vi "Simulate-Romi-Robot.vi"() -> ()   [LabVIEW 2020]
doc: "This WebSockets API example VI acts as a server for an incoming websockets connection. Receives/sends string data to the connected client."
uses:
  <vilib>/Rock Robotics/WPI/Simulation/Protocol/Devices/PWM/PWM proto.ctl
  <vilib>/Rock Robotics/WPI/Simulation/Protocol/Devices/PWM/PWM data proto.ctl
  <vilib>/Rock Robotics/WPI/Simulation/Protocol/Devices/RoboRIO/RoboRIO proto.ctl
  <vilib>/Rock Robotics/WPI/Simulation/Protocol/Devices/RoboRIO/RoboRIO data proto.ctl
  <vilib>/Rock Robotics/WPI/Simulation/Protocol/Devices/DriverStation/DS proto.ctl
  <vilib>/Rock Robotics/WPI/Simulation/Protocol/Devices/DriverStation/DS data proto.ctl
  <vilib>/Rock Robotics/WPI/Simulation/Protocol/Devices/DIO/DIO proto.ctl
  <vilib>/Rock Robotics/WPI/Simulation/Protocol/Devices/DIO/DIO data proto.ctl
  <vilib>/Rock Robotics/WPI/Simulation/Protocol/Devices/Gyro/Gyro proto.ctl
  <vilib>/Rock Robotics/WPI/Simulation/Protocol/Devices/Gyro/Gyro Data proto.ctl
  <vilib>/Rock Robotics/WPI/Simulation/Protocol/Devices/Encoder/Encoder proto.ctl
  <vilib>/Rock Robotics/WPI/Simulation/Protocol/Devices/Encoder/Encoder data protoo.ctl
  <vilib>/Rock Robotics/WPI/ThirdParty/JAS_Junk/TrajLib/DIFF_DRIVE_TRAIN_SIM.ctl
  <vilib>/Rock Robotics/WPI/ThirdParty/JAS_Junk/TrajLib/LINEAR_SYSTEM.ctl
  <vilib>/Analysis/Matrix/Datatypes/RealMatrix.ctl
  <vilib>/Rock Robotics/WPI/ThirdParty/JAS_Junk/TrajLib/DCMOTOR.CTL
  <vilib>/vision/Image Controls.llb/IMAQ Image.ctl
  ROBOT_PICTURE.ctl
  <vilib>/Utility/miscctls.llb/LVBoundsTypeDef.ctl
  <vilib>/Rock Robotics/SystemInterfaces/DIO/FPGA_DIOPWMChannel.ctl
  <vilib>/Rock Robotics/WPI/Simulation/Protocol/Devices/PWM/PWM Update Ops.ctl
  <vilib>/Rock Robotics/WPI/Simulation/Protocol/Devices/RoboRIO/RoboRIO Update Ops.ctl
  <vilib>/Rock Robotics/WPI/Simulation/Protocol/Devices/DriverStation/DS Update Ops.ctl
  <vilib>/Rock Robotics/SystemInterfaces/DIO/FPGA_DIOChannel.ctl
  <vilib>/Rock Robotics/WPI/Simulation/Protocol/Devices/DIO/DIO Update Ops.ctl
  <vilib>/Rock Robotics/WPI/Simulation/Protocol/Devices/Gyro/Gyro Update Ops.ctl
  <vilib>/Rock Robotics/WPI/Simulation/Protocol/Devices/Encoder/Encoder Update Ops.ctl
  <vilib>/Rock Robotics/SystemInterfaces/Encoder/FPGA_EncoderIdx.ctl
  <vilib>/Rock Robotics/WPI/ThirdParty/JAS_Junk/TrajLib/Rotation_CreateAngle.vi
  <vilib>/Rock Robotics/WPI/ThirdParty/JAS_Junk/TrajLib/Translation_Create.vi
  <vilib>/mediamongrels ltd/websockets/websockets/websocket server/websocket server.lvclass
  C:/Program Files (x86)/National Instruments/LabVIEW 2020/vi.lib/mediamongrels ltd/websockets/websockets/websocket/websocket.lvclass
  <vilib>/picture/pixmap.llb/Flatten Pixmap.vi
  <vilib>/picture/pictutil.llb/Create Mask.vi
  <vilib>/Rock Robotics/WPI/ThirdParty/JAS_Junk/TrajLib/Trajectory_Library.lvlib
  <vilib>/Analysis/Matrix/NI_Matrix.lvlib
panel:
  in  "Tab Control":T1(tab)
  in  "Button\n    C":bool
  in  "Button\n    B":bool
  out "Yellow LED":bool
  out "Green LED":bool
  out "Red LED":bool
  in  "Button\n    A":bool
  out "RSL ON":picture
  out "ROBOT":T2
  out "RSL OFF":picture
  out "Field Picture":picture
  out "Y Pos Pixel":dbl format="%11.1f"
  out "X Pos Pixel":dbl format="%11.1f"
  out "Y Pos Inch":dbl format="%11.1f"
  out "X Pos Inch":dbl format="%11.1f"
  out "Gyro":T3={"type"="AI", "device"="", "name"="", "data"={"<init"=FALSE, ">connected"=FALSE, "<offsetX"=0.0, "<offsetY"=0.0, "<offsetZ"=0.0, ">angleX"=0.0, ">angleY"=0.0, ">angleZ"=0.0, ">rateX"=0.0, ">rateY"=0.0, ">rateZ"=0.0, "<gain"=0.0}}
  out "DIO 0":T5={"type"="DIO", "device"="", "name"="", "data"={"<init"=FALSE, "<>value"=FALSE, "<pulse_length"=0, "<input"=FALSE}}
  out "Enc Left":T7={"type"="Encoder", "device"="", "name"="", "data"={"<init"=FALSE, ">count"=0.0, ">period"=0.0, "<samples_to_avg"=0, "<offset"=0.0, "<channel_a"=0, "<channel_b"=0}}
  out "Enc Right":T7={"type"="Encoder", "device"="", "name"="", "data"={"<init"=FALSE, ">count"=0.0, ">period"=0.0, "<samples_to_avg"=0, "<offset"=0.0, "<channel_a"=0, "<channel_b"=0}}
  out "DIO 1\nIn":T5={"type"="DIO", "device"="", "name"="", "data"={"<init"=FALSE, "<>value"=FALSE, "<pulse_length"=0, "<input"=FALSE}}
  out "DIO 2\nIn":T5={"type"="DIO", "device"="", "name"="", "data"={"<init"=FALSE, "<>value"=FALSE, "<pulse_length"=0, "<input"=FALSE}}
  out "PWM 0":T9
  out "PWM 1":T9
  out "DIO 1\nOut":T5={"type"="DIO", "device"="", "name"="", "data"={"<init"=FALSE, "<>value"=FALSE, "<pulse_length"=0, "<input"=FALSE}}
  out "DIO 2\nOut":T5={"type"="DIO", "device"="", "name"="", "data"={"<init"=FALSE, "<>value"=FALSE, "<pulse_length"=0, "<input"=FALSE}}
  out "DIO 3":T5={"type"="DIO", "device"="", "name"="", "data"={"<init"=FALSE, "<>value"=FALSE, "<pulse_length"=0, "<input"=FALSE}}
  out "roboRIO new":T11={"type"="roboRIO", "device"="", "name"="", "data"={">fpga_button"=FALSE, ">vin_voltage"=0.0, ">vin_current"=0.0, ">6v_voltage"=0.0, ">6v_current"=0.0, ">6v_active"=FALSE, ">6v_faults"=0.0, ">5v_voltage"=0.0, ">5v_current"=0.0, ">5v_active"=FALSE, ">5v_faults"=0.0, ">3v3_voltage"=0.0, ">3v3_current"=0.0, ">3v3_active"=FALSE, ">3v3_faults"=0.0}}
  out "Driverstation new":T13={"type"="Driverstation", "device"="", "name"="", "data"={">enabled"=FALSE, ">autonomous"=FALSE, ">test"=FALSE, ">estop"=FALSE, ">fms"=FALSE, ">ds"=FALSE, "<match_time"=0.0, ">station"="", ">game_data"=""}}
  out "Request URI":string
  out "HTTP Headers":variant
  out "Stop Sim":bool
  out "Battery Voltage VDC":dbl format="%18.2f"
  out "Sim Heading":dbl format="%19.3f"
  out "Edges/Feet":dbl
  out "out DiffDriveTrainSim":T15 {"m_Motor"."Jr_KgM2" format="%13.5p"; "m_Motor"."L_H" format="%13.5p"; "m_Motor"."Kt_NMPerAmp" format="%13.5p"; "m_Motor"."KvINV_RadPerSecPerVolt" format="%13.5p"; "m_Motor"."R_Ohms" format="%13.5p"; "m_Motor"."FreeSpeed_RadPerSec" format="%13.5p"; "m_Motor"."FreeCurrent_Amps" format="%13.5p"; "m_Motor"."StallCurrent_Amps" format="%13.5p"; "m_Motor"."StallTorque_NM" format="%13.5p"; "m_Motor"."nominalVoltage_Volts" format="%13.5p"}
  out "Speed Left":dbl format="%13.2f"
  out "Speed Right":dbl format="%13.2f"
  out "Amps":dbl
  out "PWM 0 Rate":dbl format="%19.3f"
  out "PWM 1 Rate":dbl format="%19.3f"
  out "FIeld Image":T19
  # "Robot Position"
  # "<States, 1>"
  # "<Outputs, 1>"
  # "<Inputs, 1>"
  # "<Outputs, 1>"
  # "<States,States>"
  # "<States,Inputs>"
  # "<Outputs,States>"
  # "<Outputs,Inputs>"
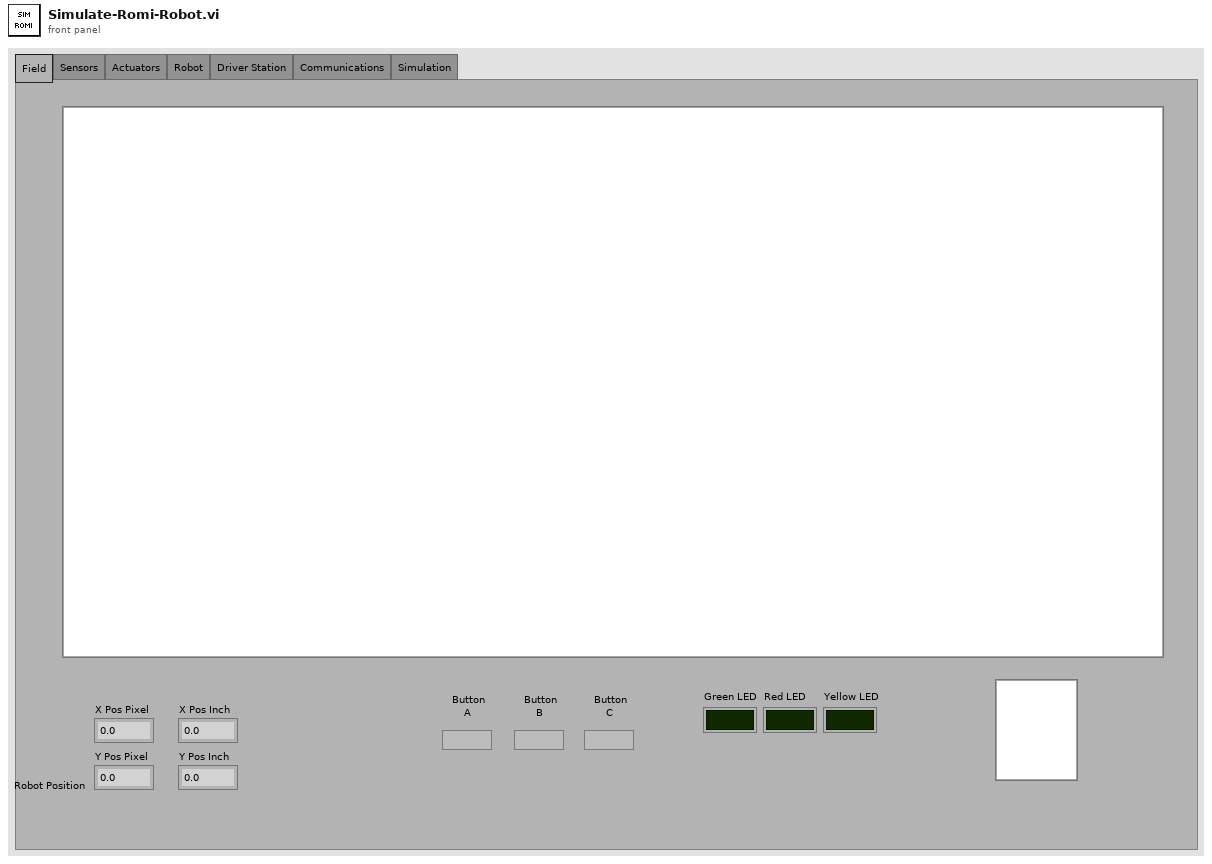
[diagram p1: front panel]
types:
  T1 = enum32{"Field", "Sensors", "Actuators", "Robot", "Driver Station", "Communications", "Simulation"}
  T2 = typedef "ROBOT_PICTURE.ctl" = picture
  T3 = typedef "Gyro proto.ctl" = cluster{"type":string, "device":string, "name":string, "data":T4}
  T4 = typedef "Gyro Data proto.ctl" = cluster{"<init":bool, ">connected":bool, "<offsetX":dbl, "<offsetY":dbl, "<offsetZ":dbl, ">angleX":dbl, ">angleY":dbl, ">angleZ":dbl, ">rateX":dbl, ">rateY":dbl, ">rateZ":dbl, "<gain":dbl}
  T5 = typedef "DIO proto.ctl" = cluster{"type":string, "device":string, "name":string, "data":T6}
  T6 = typedef "DIO data proto.ctl" = cluster{"<init":bool, "<>value":bool, "<pulse_length":i32, "<input":bool}
  T7 = typedef "Encoder proto.ctl" = cluster{"type":string, "device":string, "name":string, "data":T8}
  T8 = typedef "Encoder data protoo.ctl" = cluster{"<init":bool, ">count":dbl, ">period":dbl, "<samples_to_avg":i32, "<offset":dbl, "<channel_a":i32, "<channel_b":i32}
  T9 = typedef "PWM proto.ctl" = cluster{"type":string, "device":string, "name":string, "data":T10}
  T10 = typedef "PWM data proto.ctl" = cluster{"<init":bool, "<speed":dbl, "<position":dbl, "<raw":dbl, "<period_scale":dbl, "<zero_latch":bool, "<servo range":dbl}
  T11 = typedef "RoboRIO proto.ctl" = cluster{"type":string, "device":string, "name":string, "data":T12}
  T12 = typedef "RoboRIO data proto.ctl" = cluster{">fpga_button":bool, ">vin_voltage":dbl, ">vin_current":dbl, ">6v_voltage":dbl, ">6v_current":dbl, ">6v_active":bool, ">6v_faults":dbl, ">5v_voltage":dbl, ">5v_current":dbl, ">5v_active":bool, ">5v_faults":dbl, ">3v3_voltage":dbl, ">3v3_current":dbl, ">3v3_active":bool, ">3v3_faults":dbl}
  T13 = typedef "DS proto.ctl" = cluster{"type":string, "device":string, "name":string, "data":T14}
  T14 = typedef "DS data proto.ctl" = cluster{">enabled":bool, ">autonomous":bool, ">test":bool, ">estop":bool, ">fms":bool, ">ds":bool, "<match_time":dbl, ">station":string, ">game_data":string}
  T15 = typedef "Trajectory_Library.lvlib/DIFF_DRIVE_TRAIN_SIM.ctl" = cluster{"m_Plant":T16, "m_X":T17, "m_Y":T17, "m_U":T17, "MeasureStdDev":T17, "m_Motor":T18, "m_OriginalGearing":dbl, "m_CurrentGearing":dbl, "m_WheelRadius_M":dbl, "m_RB":dbl}
  T16 = typedef "Trajectory_Library.lvlib/LINEAR_SYSTEM.ctl" = cluster{"m_A":T17, "m_B":T17, "m_C":T17, "m_D":T17, "States":i32, "Inputs":i32, "Outputs":i32}
  T17 = typedef "NI_Matrix.lvlib/RealMatrix.ctl" = dbl[][]
  T18 = typedef "Trajectory_Library.lvlib/DCMOTOR.CTL" = cluster{"nominalVoltage_Volts":dbl, "StallTorque_NM":dbl, "StallCurrent_Amps":dbl, "FreeCurrent_Amps":dbl, "FreeSpeed_RadPerSec":dbl, "R_Ohms":dbl, "KvINV_RadPerSecPerVolt":dbl, "Kt_NMPerAmp":dbl, "L_H":dbl, "Jr_KgM2":dbl}
  T19 = typedef "IMAQ Image.ctl" = refnum<image>
  T20 = typedef "LVBoundsTypeDef.ctl" = cluster{"Width":u32, "Height":u32}
  T21 = typedef "Image Type" = u32
  T22 = typedef "imagedata.ctl" = cluster{"image type":i32, "image depth":i32, "image":u8[], "mask":u8[], "colors":u32[], "Rectangle":cluster{"left":i16, "top":i16, "right":i16, "bottom":i16}}
  T23 = typedef "TrajectoryUtils_Field_Info.ctl" = cluster{"FIeld_File_Name":string, "Top_Left_X":i32, "Top_Left_Y":i32, "Bottom_Right_X":i32, "Bottom_Right_Y":i32, "Field_Size_X":dbl, "Field_Size_Y":dbl, "FIeld_Size_Units":string}
  T24 = typedef "Trajectory_Library.lvlib/POSE2D.ctl" = cluster{"TRANSLATION":T25, "ROTATION":T26}
  T25 = typedef "Trajectory_Library.lvlib/TRANSLATION2D.ctl" = cluster{"X":dbl, "Y":dbl}
  T26 = typedef "Trajectory_Library.lvlib/ROTATION2D.ctl" = cluster{"VALUE":dbl, "COS":dbl, "SIN":dbl}
  T27 = typedef "Rotated_Picture_TypeDef.ctl" = cluster{"ONE-8-bit pixmap":u8[][], "Two-Array":cdb[][], "Three-Numeric":i32, "Four-Numeric":i32, "Five-Numeric":cdb, "Six-colors":u32[], "Seven-new element/subarray":u32, "Eight-Cluster":cluster{"[0]":i32, "[1]":i32}}
  T28 = typedef "Encoder Update Ops.ctl" = enum16{"set init", "set count", "set period", "set reset", "set samples_to_avg", "get", "delete", "JSON update", "set name", "transmit initial", "reset", "set channel_a", "set channel_b"}
  T29 = typedef "FPGA_EncoderIdx.ctl" = enum8{"Enc 0", "Enc 1", "Enc 2", "Enc 3", "Enc 4", "Enc 5", "Enc 6", "Enc 7", "Invalid"}
  T30 = typedef "Gyro Update Ops.ctl" = enum16{"get", "delete", "JSON update", "set  name", "transmit initial", "reset", "set init", "set offsetX", "set offsetY", "set offsetZ", "set gain"}
  T31 = typedef "FPGA_DIOChannel.ctl" = enum8{"DIO 0", "DIO 1", "DIO 2", "DIO 3", "DIO 4", "DIO 5", "DIO 6", "DIO 7", "DIO 8", "DIO 9", "DIO MXP 0", "DIO MXP 1", "DIO MXP 2", "DIO MXP 3", "DIO MXP 4", "DIO MXP 5", "DIO MXP 6", "DIO MXP 7", "DIO MXP 8", "DIO MXP 9", "DIO MXP 10", "DIO MXP 11", "DIO MXP 12", "DIO MXP 13", "DIO MXP 14", "DIO MXP 15", "SPI Port CS1", "SPI Port CS2", "SPI Port CS3", "SPI Port MISO", "SPI Port MOSI", "Invalid"}
  T32 = typedef "DIO Update Ops.ctl" = enum16{"set init", "set value", "set pulse_length", "set input", "get", "delete", "JSON update", "set name", "transmit initial", "reset"}
  T33 = typedef "DS Update Ops.ctl" = enum16{"set enabled", "set autonomous", "set test", "set estop", "set fms", "set ds", "set control word", "set match_time", "set station", "set game data", "JSON update", "set name", "get", "transmit initial", "reset"}
  T34 = typedef "RoboRIO Update Ops.ctl" = enum16{"get", "JSON update", "set name", "transmit initial", "set fpga_button", "set vin_voltage", "set vin_current", "set 6v_voltage", "set 6v_current", "set 6v_active", "set 6v_faults", "set 5v_voltage", "set 5v_current", "set 5v_active", "set 5v_faults", "set 3v3_voltage", "set 3v3_current", "set 3v3_active", "set 3v3_faults", "reset"}
  T35 = typedef "FPGA_DIOPWMChannel.ctl" = enum8{"PWM 0", "PWM 1", "PWM 2", "PWM 3", "PWM 4", "PWM 5", "PWM 6", "PWM 7", "PWM 8", "PWM 9", "PWM MXP 0", "PWM MXP 1", "PWM MXP 2", "PWM MXP 3", "PWM MXP 4", "PWM MXP 5", "PWM MXP 6", "PWM MXP 7", "PWM MXP 8", "PWM MXP 9", "Invalid"}
  T36 = typedef "PWM Update Ops.ctl" = enum16{"set init", "set speed", "set position", "set raw", "set  period_scale", "set zero_latch", "set angular range", "get", "delete", "JSON update", "set name", "transmit initial", "reset"}
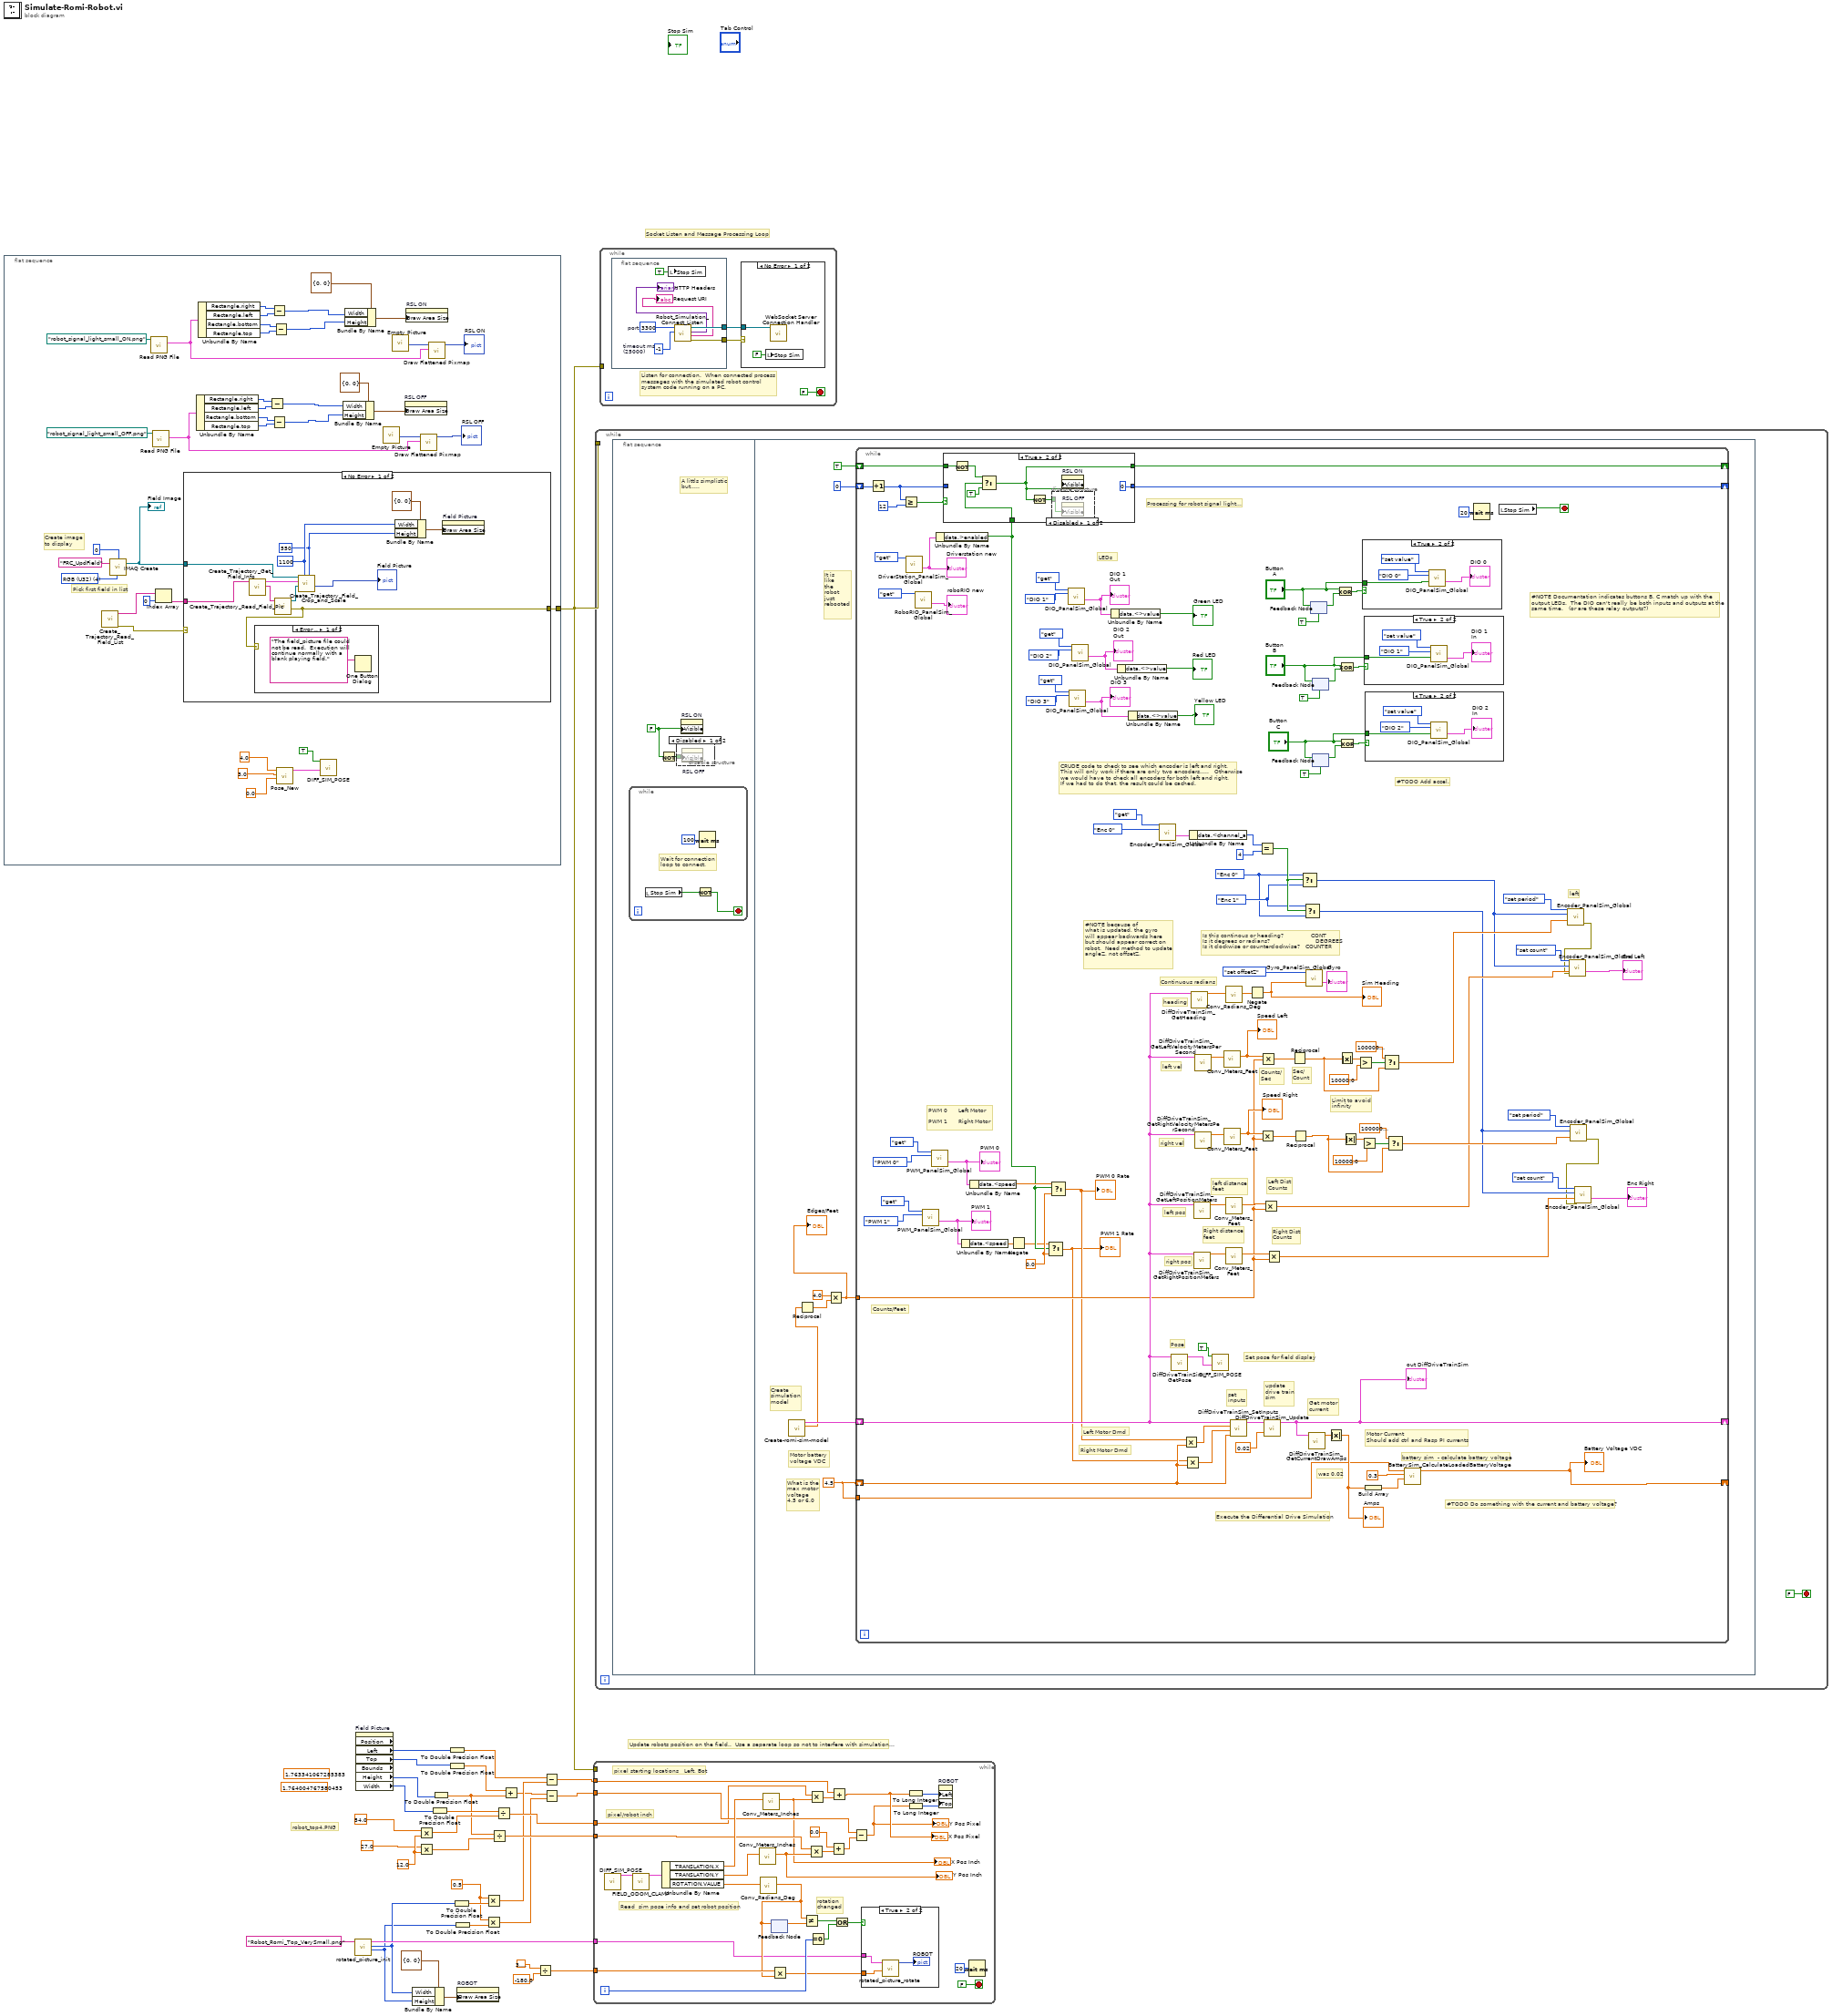
[diagram p0: block diagram]
diagram:
  w9 = 0.5
  (unwired) 1.764004767580453
  (unwired) 1.763341067285383
  w27 = 12.0 ("y")
  # "Update robots position on the field..  Use a separate loop so not to interfere with simulation..."
  # "robot_top4.PNG"
  # "Socket Listen and Message Processing Loop"
  n1 = flat-sequence {
    tunnel: [w43] -> w28
    frame #0 {
      w68 = T21 4 items=["Grayscale (U8)", "Grayscale (I16)", "Grayscale (SGL)", "Complex (CSG)", "RGB (U32)", "HSL (U32)", "RGB (U64)", "Grayscale (U16)"] ("Image Type")
      # "Pick first field in list"
      # "Create image \nto display"
      n2 = call "Create_Trajectory_Read_Field_List.vi"() -> ("error out"=w66:errorcluster, "section names"=w67:string[])  [unwired: 10 in]
      n3 = call "IMAQ Create"("Border Size"=0, "Image Name"="FRC_UpdField", "Image Type"=w68) -> ("New Image"=w65:T19)  [unwired: 2 in, 1 out]
      "FIeld Image" <- w65
      n4 = call <vilib>:"Read PNG File.vi"("path to PNG file"=path "robot_signal_light_small_ON.png") -> ("image data"=w54:T22)  [unwired: 8 in, 2 out]
      n5 = call <vilib>:"Read PNG File.vi"("path to PNG file"=path "robot_signal_light_small_OFF.png") -> ("image data"=w61:T22)  [unwired: 8 in, 2 out]
      n6 = Index Array(array=w67, index=0) -> (element=w64:string)
      n7 = case shown="No Error" w66 {
        selector: w66 -> [_ w84]
        tunnel: w65 -> [w79 _]
        tunnel: [w78 w84] -> w43
        tunnel: w64 -> [w77 _]
        frame No Error {
          w72 = 550 ("Disp Y Size Pixel")
          w73 = 1100 ("Disp X Size Pixel")
          n8 = call "Create_Trajectory_Get_Field_Info.vi"("Field Selector"=w77) -> ("File"=w82:string, "input cluster"=w81:T23)  [unwired: 9 in]
          n9 = call "Create_Trajectory_Read_Field_Pic.vi"("file name"=w82) -> ("Image Error"=w78:errorcluster, "Image Data"=w80:T19)  [unwired: 7 in, 2 out]
          n10 = case shown="Error .." w78 {
            frame Error {
              n11 = One Button Dialog(message="The field_picture file could not be read.  Execution will continue normally with a blank playing field.") -> ()  [unwired: 1 in, 1 out]
            }
            frame No Error {
            }
          }
          n12 = call "Create_Trajectory_Field_Crop_and_Scale.vi"("Disp Y Size Pixel"=w72, "Disp X Size Pixel"=w73, "Field Image"=w80, "field Info"=w81, "Display Image"=w79) -> ("Cropped Field Picture Out"=→"Field Picture":picture)  [unwired: 4 in, 2 out]
          n13 = Bundle By Name(cluster=T20 {"Width"=0, "Height"=0} ("Draw Area Size"), "Width"=w73, "Height"=w72) -> (w74:T20)
          n14 = property on="Field Picture" class="Pict"("Draw Area Size"=w74) -> ()  [unwired: 2 in, 2 out]
        }
        frame Error {
        }
      }
      n15 = Unbundle By Name(w61) -> ("Rectangle.right"=w57:i16, "Rectangle.left"=w58:i16, "Rectangle.bottom"=w56:i16, "Rectangle.top"=w59:i16)
      n16 = Unbundle By Name(w54) -> ("Rectangle.right"=w49:i16, "Rectangle.left"=w50:i16, "Rectangle.bottom"=w48:i16, "Rectangle.top"=w51:i16)
      n17 = Subtract(x=w57, y=w58) -> (x-y=w35:i16)
      n18 = Subtract(x=w49, y=w50) -> (x-y=w37:i16)
      n19 = Subtract(x=w56, y=w59) -> (x-y=w34:i16)
      n20 = Subtract(x=w48, y=w51) -> (x-y=w36:i16)
      n21 = call <vilib>:"Pose_New.vi"("Heading"=0.0, "Y"=3.0, "X"=4.0) -> ("out POSe"=w41:T24)  [unwired: 8 in]
      n22 = call "DIFF_SIM_POSE.vi"("in Sim Pose"=w41, "WRITE"=TRUE) -> ()  [unwired: 9 in, 1 out]
      n23 = Bundle By Name(cluster=T20 {"Width"=0, "Height"=0} ("Draw Area Size"), "Width"=w35, "Height"=w34) -> (w63:T20)
      n24 = Bundle By Name(cluster=T20 {"Width"=0, "Height"=0} ("Draw Area Size"), "Width"=w37, "Height"=w36) -> (w52:T20)
      n25 = call "Empty Picture"() -> ("empty picture"=w60:picture)
      n26 = call "Empty Picture"() -> ("empty picture"=w53:picture)
      n27 = property on="RSL OFF" class="Pict"("Draw Area Size"=w63) -> ()  [unwired: 2 in, 2 out]
      n28 = property on="RSL ON" class="Pict"("Draw Area Size"=w52) -> ()  [unwired: 2 in, 2 out]
      n29 = call <vilib>:"Draw Flattened Pixmap.vi"("image data"=w61, "picture"=w60) -> ("new picture"=→"RSL OFF":picture)  [unwired: 7 in]
      n30 = call <vilib>:"Draw Flattened Pixmap.vi"("image data"=w54, "picture"=w53) -> ("new picture"=→"RSL ON":picture)  [unwired: 7 in]
    }
  }
  n31 = call "rotated_picture_init.vi"("Picture FIle Name"="Robot_Romi_Top_VerySmall.png" ("name or relative path")) -> ("Height"=w1:i16, "Width"=w2:i16, "RotatedPictureInfo"=w29:T27)  [unwired: 7 in, 1 out]
  n32 = property on="Field Picture" class="Pict" props=["Position", "Left", "Top", "Bounds", "Height", "Width"]() -> ("Left"=w24:i32, "Top"=w23:i32, "Height"=w22:u32, "Width"=w21:u32)  [unwired: 2 in, 4 out]
  n33 = Bundle By Name(cluster=T20 {"Width"=0, "Height"=0} ("Draw Area Size"), "Width"=w2, "Height"=w1) -> (w4:T20)
  n34 = Multiply(x=54.0, y=w27) -> (x*y=w18:dbl)
  n35 = Multiply(x=27.0, y=w27) -> (x*y=w15:dbl)
  n36 = To Double Precision Float(number=w21) -> (double precision float=w19:dbl)
  n37 = To Double Precision Float(number=w22) -> (double precision float=w16:dbl)
  n38 = To Double Precision Float(number=w24) -> (double precision float=w8:dbl)
  n39 = To Double Precision Float(number=w23) -> (double precision float=w20:dbl)
  n40 = To Double Precision Float(number=w2) -> (double precision float=w11:dbl)
  n41 = To Double Precision Float(number=w1) -> (double precision float=w10:dbl)
  n42 = property on="ROBOT" class="Pict (strict)"("Draw Area Size"=w4) -> ()  [unwired: 2 in, 2 out]
  n43 = Multiply(x=w9, y=w11) -> (x*y=w7:dbl)
  n44 = Multiply(x=w9, y=w10) -> (x*y=w5:dbl)
  n45 = Divide(x=w16, y=w15) -> (x/y=w14:dbl)
  n46 = Divide(x=w19, y=w18) -> (x/y=w17:dbl)
  n47 = Add(x=w20, y=w16) -> (x+y=w6:dbl)
  n48 = Divide(x=3.141592653589793, y=-180.0 ("value")) -> (x/y=w33:dbl)
  n49 = Subtract(x=w8, y=w7) -> (x-y=w13:dbl)
  n50 = Subtract(x=w6, y=w5) -> (x-y=w12:dbl)
  n51 = while {
    tunnel: w33 -> [w114]
    tunnel: w29 -> [w97]
    tunnel: w28 -> [_]
    tunnel: w13 -> [w94]
    tunnel: w12 -> [w93]
    tunnel: w17 -> [w92]
    tunnel: w14 -> [w91]
    i -> [w103]
    stop <- FALSE stop-if-true
    # "pixel starting locations   Left, Bot"
    # "Read  sim pose info and set robot position"
    # "pixel/robot inch"
    # "rotation\nchanged"
    n52 = call "DIFF_SIM_POSE.vi"() -> ("out Sim Pose"=w96:T24)  [unwired: 11 in]
    n53 = call "FIELD_ODOM_CLAMP.vi"("in Sim Pose"=w96) -> ("out Sim Pose"=w95:T24)  [unwired: 10 in]
    n54 = Unbundle By Name(w95) -> ("TRANSLATION.X"=w102:dbl, "TRANSLATION.Y"=w101:dbl, "ROTATION.VALUE"=w99:dbl)
    n55 = call <vilib>:"Conv_Meters_Inches.vi"("Meters"=w101) -> ("Inches"=w86:dbl)  [unwired: 10 in]
    "Y Pos Inch" <- w86
    n56 = call <vilib>:"Conv_Radians_Deg.vi"("Radians"=w99) -> ("Degrees"=w100:dbl)  [unwired: 10 in]
    n57 = call <vilib>:"Conv_Meters_Inches.vi"("Meters"=w102) -> ("Inches"=w85:dbl)  [unwired: 10 in]
    "X Pos Inch" <- w85
    n58 = feedback-in #1(w100) -> ()
    n59 = feedback #1() -> (w111:dbl)  [unwired: 1 in]
    n60 = Multiply(x=w114, y=w100) -> (x*y=w98:dbl)
    n61 = Not Equal?(x=w100, y=w111) -> (x != y?=w105:bool)
    n62 = Multiply(x=w91, y=w86) -> (x*y=w109:dbl)
    n63 = Multiply(x=w92, y=w85) -> (x*y=w110:dbl)
    n64 = Equal To 0?(x=w103) -> (x = 0?=w104:bool)
    n65 = Add(x=0.0, y=w109) -> (x+y=w107:dbl)
    n66 = Add(x=w94, y=w110) -> (x+y=w88:dbl)
    "X Pos Pixel" <- w88
    n67 = Or(x=w105, y=w104) -> (x .or. y?=w106:bool)
    n68 = Subtract(x=w93, y=w107) -> (x-y=w87:dbl)
    "Y Pos Pixel" <- w87
    n69 = case shown="True" w106 {
      tunnel: w98 -> [_ w115]
      tunnel: w97 -> [_ w116]
      frame False {
      }
      frame True {
        n70 = call "rotated_picture_rotate.vi"("Angle"=w115, "RotatedPictureInfo"=w116) -> ("new picture"=→"ROBOT":picture)  [unwired: 9 in]
      }
    }
    n71 = To Long Integer(number=w88) -> (32bit integer=w90:i32)
    n72 = To Long Integer(number=w87) -> (32bit integer=w89:i32)
    n73 = property on="ROBOT" class="Pict (strict)"("Left"=w90, "Top"=w89) -> ()  [unwired: 2 in, 2 out]
    n74 = Wait (ms)(milliseconds to wait=u32 20) -> ()  [unwired: 1 out]
  }
  n75 = while {
    tunnel: w28 -> [_]
    stop <- FALSE stop-if-true
    n76 = flat-sequence {
      frame #0 {
        w119 = FALSE ("Visible")
        # "A littls simplistic\nbut....."
        n77 = while {
          stop <- w122 stop-if-true
          # "Wait for connection\nloop to connect."
          n78 = local read "Stop Sim"() -> (w123:bool)
          n79 = Not(x=w123) -> (.not. x?=w122:bool)
          n80 = Wait (ms)(milliseconds to wait=u32 100) -> ()  [unwired: 1 out]
        }
        n81 = Not(x=w119) -> (.not. x?=w120:bool)
        n82 = disable-structure shown="Disabled" {
          disable-tunnel: w120 -> [w121 _]
          frame Disabled {
            n83 = property on="RSL OFF" class="Pict"("Visible"=w121) -> ()  [unwired: 2 in, 2 out]
          }
          frame Enabled {
          }
        }
        n84 = property on="RSL ON" class="Pict"("Visible"=w119) -> ()  [unwired: 2 in, 2 out]
      }
      frame #1 {
        w129 = 4.5 ("Voltage")
        # "Create\nsimulation\nmodel"
        # "Motor battery\nvoltage VDC"
        # "What is the\nmax motor\nvoltage\n4.5 or 6.0"
        # "It is\nlike\nthe \nrobot \njust\nrebooted"
        n85 = call "Create-romi-sim-model.vi"() -> ("Encoder Ft/Count"=w126:dbl, "out DiffDriveTrainSim"=w130:T15)  [unwired: 10 in]
        n86 = Reciprocal(x=w126) -> (1/x=w127:dbl)
        n87 = Multiply(x=4.0, y=w127) -> (x*y=w125:dbl)
        "Edges/Feet" <- w125
        n88 = while {
          shift-right: [w208] -> _
          shift-left: 0 -> [w213]
          shift-right: [w210] -> _
          shift-left: TRUE -> [w211]
          shift-right: [w191] -> _
          shift-left: w130 -> [w192]
          shift-right: [w188] -> _
          shift-left: w129 -> [w190]
          tunnel: w129 -> [w189]
          tunnel: w125 -> [w180]
          stop <- w215 stop-if-true
          w166 = FPGA_EncoderIdx."Enc 1" ("EncoderIndex")
          w165 = FPGA_EncoderIdx."Enc 0" ("EncoderIndex")
          w174 = 0.0 ("f")
          # "was 0.02"
          # "LEDs"
          # "#NOTE Documentation indicates buttons B, C match up with the\noutput LEDs.  The DIO can't really be both inputs and outputs at the\nsame time.   (or are these relay outputs?)"
          # "#NOTE because of\nwhat is updated, the gyro\nwill appear backwards here\nbut should appear correct on\nrobot.  Need method to update\nangleZ, not offsetZ."
          # "#TODO Add accel."
          # "left"
          # "CRUDE code to check to see which encoder is left and right.\nThis will only work if there are only two encoders.....   Otherwise\nwe would have to check all encoders for both left and right.\nIf we had to do that, the result could be cached."
          # "#TODO Do something with the current and battery voltage?"
          # "Right Dist\nCounts"
          # "Left Dist\nCounts"
          # "Is this continous or heading?               CONT\nIs it degrees or radians?                         DEGREES\nIs it clockwise or counterclockwise?   COUNTER"
          # "Sec/\nCount"
          # "Limit to avoid\ninfinity"
          # "Counts/\nSec"
          # "Counts/Feet"
          # "Get motor\ncurrent"
          # "Set pose for field display"
          # "PWM 0      Left Motor\n\nPWM 1      Right Motor"
          # "Motor Current\nShould add ctrl and Rasp PI currents"
          # "Right Motor Dmd"
          # "Left Motor Dmd"
          # "Continuous radians"
          # "Right distance\nfeet"
          # "left distance\nfeet"
          # "Execute the Differential Drive Simulation"
          # "heading"
          # "left pos"
          # "right pos"
          # "right vel"
          # "left vel"
          # "Pose"
          # "update\ndrive train\nsim"
          # "set\ninputs"
          # "battery sim  - calculate battery voltage"
          # "Processing for robot signal light..."
          n89 = Increment(x=w213) -> (x+1=w209:i32)
          n90 = Greater Or Equal?(x=w209, y=12) -> (x >= y?=w207:bool)
          n91 = call <vilib>:"DriverStation_PanelSim_Global.vi"("menu"=DS_Update_Ops."get") -> ("Driverstation new"=w214:T13)  [unwired: 13 in, 1 out]
          "Driverstation new" <- w214
          n92 = call <vilib>:"RoboRIO_PanelSim_Global.vi"("Menu"=RoboRIO_Update_Ops."get") -> ("roboRIO new"=→"roboRIO new":T11)  [unwired: 13 in, 1 out]
          n93 = call <vilib>:"PWM_PanelSim_Global.vi"("menu"=PWM_Update_Ops."get", "PWMChannel"=FPGA_DIOPWMChannel."PWM 1") -> ("Value get"=w239:T9)  [unwired: 12 in, 1 out]
          "PWM 1" <- w239
          n94 = call <vilib>:"PWM_PanelSim_Global.vi"("menu"=PWM_Update_Ops."get", "PWMChannel"=FPGA_DIOPWMChannel."PWM 0") -> ("Value get"=w242:T9)  [unwired: 12 in, 1 out]
          "PWM 0" <- w242
          n95 = Unbundle By Name(w214) -> ("data.>enabled"=w173:bool)
          n96 = case shown="True" w207 {
            tunnel: w211 -> [w259 w266]
            tunnel: [w259 w261] -> w210
            tunnel: w209 -> [w258 _]
            tunnel: [w258 0] -> w208
            tunnel: w173 -> [_ w264]
            frame False {
            }
            frame True {
              n97 = Not(x=w266) -> (.not. x?=w265:bool)
              n98 = Select(t=w265, s=w264, f=TRUE) -> (s? t:f=w261:bool)
              n99 = Not(x=w261) -> (.not. x?=w262:bool)
              n100 = disable-structure shown="Disabled" {
                disable-tunnel: w262 -> [w267 _]
                frame Disabled {
                  n101 = property on="RSL OFF" class="Pict"("Visible"=w267) -> ()  [unwired: 2 in, 2 out]
                }
                frame Enabled {
                }
              }
              n102 = property on="RSL ON" class="Pict"("Visible"=w261) -> ()  [unwired: 2 in, 2 out]
            }
          }
          n103 = Unbundle By Name(w239) -> ("data.<speed"=w161:dbl)
          n104 = Unbundle By Name(w242) -> ("data.<speed"=w175:dbl)
          n105 = Negate(x=w161) -> (-x=w160:dbl)
          n106 = Select(t=w160, s=w173, f=w174) -> (s? t:f=w176:dbl)
          "PWM 1 Rate" <- w176
          n107 = Select(t=w175, s=w173, f=w174) -> (s? t:f=w177:dbl)
          "PWM 0 Rate" <- w177
          n108 = call <vilib>:"DIO_PanelSim_Global.vi"("menu"=DIO_Update_Ops."get", "DIO Channel"=FPGA_DIOChannel."DIO 1") -> ("DIO new"=w228:T5)  [unwired: 12 in, 1 out]
          "DIO 1\nOut" <- w228
          n109 = call <vilib>:"DIO_PanelSim_Global.vi"("menu"=DIO_Update_Ops."get", "DIO Channel"=FPGA_DIOChannel."DIO 3") -> ("DIO new"=w148:T5)  [unwired: 12 in, 1 out]
          "DIO 3" <- w148
          n110 = call <vilib>:"DIO_PanelSim_Global.vi"("menu"=DIO_Update_Ops."get", "DIO Channel"=FPGA_DIOChannel."DIO 2") -> ("DIO new"=w227:T5)  [unwired: 12 in, 1 out]
          "DIO 2\nOut" <- w227
          n111 = Unbundle By Name(w228) -> ("data.<>value"=→"Green LED":bool)
          n112 = Unbundle By Name(w227) -> ("data.<>value"=→"Red LED":bool)
          n113 = Unbundle By Name(w148) -> ("data.<>value"=→"Yellow LED":bool)
          n114 = call <vilib>:"Encoder_PanelSim_Global.vi"("menu"=Encoder_Update_Ops."get", "EncoderIndex"=FPGA_EncoderIdx."Enc 0") -> ("Encoder new"=w170:T7)  [unwired: 12 in, 1 out]
          n115 = call <vilib>:"DiffDriveTrainSim_GetPose.vi"("DiffDriveTrainSim"=w192) -> ("Pose"=w200:T24)  [unwired: 10 in]
          n116 = Multiply(x=w177, y=w190) -> (x*y=w198:dbl)
          n117 = Multiply(x=w176, y=w190) -> (x*y=w197:dbl)
          n118 = Unbundle By Name(w170) -> ("data.<channel_a"=w169:i32)
          n119 = call <vilib>:"DiffDriveTrainSim_GetHeading.vi"("DiffDriveTrainSim"=w192) -> ("Heading"=w151:dbl)  [unwired: 10 in]
          n120 = call <vilib>:"DiffDriveTrainSim_GetLeftPositionMeters.vi"("DiffDriveTrainSim"=w192) -> ("LeftPosition_Meters"=w193:dbl)  [unwired: 10 in]
          n121 = call <vilib>:"DiffDriveTrainSim_GetRightPositionMeters.vi"("DiffDriveTrainSim"=w192) -> ("RightPosition_Meters"=w196:dbl)  [unwired: 10 in]
          n122 = call <vilib>:"DiffDriveTrainSim_GetRightVelocityMetersPerSecond.vi"("DiffDriveTrainSim"=w192) -> ("RightVel_M_Per_Sec"=w195:dbl)  [unwired: 10 in]
          n123 = call <vilib>:"DiffDriveTrainSim_GetLeftVelocityMetersPerSecond.vi"("DiffDriveTrainSim"=w192) -> ("LeftVelocity_M_Per_Sec"=w194:dbl)  [unwired: 10 in]
          n124 = call "DIFF_SIM_POSE.vi"("in Sim Pose"=w200, "WRITE"=TRUE) -> ()  [unwired: 9 in, 1 out]
          n125 = call <vilib>:"Conv_Meters_Feet.vi"("Meters"=w194) -> ("Feet"=w162:dbl)  [unwired: 10 in]
          "Speed Left" <- w162
          n126 = call <vilib>:"Conv_Meters_Feet.vi"("Meters"=w195) -> ("Feet"=w187:dbl)  [unwired: 10 in]
          "Speed Right" <- w187
          n127 = call <vilib>:"Conv_Radians_Deg.vi"("Radians"=w151) -> ("Degrees"=w150:dbl)  [unwired: 10 in]
          n128 = call <vilib>:"Conv_Meters_Feet.vi"("Meters"=w196) -> ("Feet"=w182:dbl)  [unwired: 10 in]
          n129 = call <vilib>:"Conv_Meters_Feet.vi"("Meters"=w193) -> ("Feet"=w181:dbl)  [unwired: 10 in]
          n130 = call <vilib>:"DiffDriveTrainSim_SetInputs.vi"("BatteryVoltage"=w190, "Right_Volts"=w197, "Left_Volts"=w198, "in DiffDriveTrainSim"=w192) -> ("out DiffDriveTrainSim"=w206:T15)  [unwired: 6 in, 1 out]
          n131 = Negate(x=w150) -> (-x=w149:dbl)
          "Sim Heading" <- w149
          n132 = Equal?(x=w169, y=4) -> (x = y?=w167:bool)
          n133 = Multiply(x=w187, y=w180) -> (x*y=w186:dbl)
          n134 = Multiply(x=w162, y=w180) -> (x*y=w185:dbl)
          n135 = Multiply(x=w181, y=w180) -> (x*y=w179:dbl)
          n136 = call <vilib>:"DiffDriveTrainSim_Update.vi"("dT_Seconds"=0.02, "in DiffDriveTrainSim"=w206) -> ("out DiffDriveTrainSim"=w191:T15)  [unwired: 8 in, 1 out]
          "out DiffDriveTrainSim" <- w191
          n137 = Multiply(x=w182, y=w180) -> (x*y=w178:dbl)
          n138 = Reciprocal(x=w185) -> (1/x=w183:dbl)
          n139 = Reciprocal(x=w186) -> (1/x=w184:dbl)
          n140 = Select(t=w165, s=w167, f=w166) -> (s? t:f=w164:T29)
          n141 = Select(t=w166, s=w167, f=w165) -> (s? t:f=w163:T29)
          n142 = call <vilib>:"Gyro_PanelSim_Global.vi"("Menu"=Gyro_Update_Ops."set offsetZ", "Numeric Value"=w149) -> ("Value out"=→"Gyro":T3)  [unwired: 12 in, 1 out]
          n143 = call <vilib>:"DiffDriveTrainSim_GetCurrentDrawAmps.vi"("DiffDriveTrainSim"=w191) -> ("TotalCurrent_Amps"=w202:dbl)  [unwired: 10 in]
          n144 = feedback-in #2("Button\n    A") -> ()
          n145 = feedback #2(TRUE) -> (w146:bool)
          n146 = feedback #3(TRUE) -> (w143:bool)
          n147 = feedback-in #3("Button\n    B") -> ()
          n148 = feedback #4(TRUE) -> (w140:bool)
          n149 = feedback-in #4("Button\n    C") -> ()
          n150 = Absolute Value(x=w202) -> (abs(x)=w199:dbl)
          "Amps" <- w199
          n151 = Exclusive Or(1:w146, 2:"Button\n    A") -> (0:w145:bool)
          n152 = Exclusive Or(1:w143, 2:"Button\n    B") -> (0:w142:bool)
          n153 = Absolute Value(x=w183) -> (abs(x)=w225:dbl)
          n154 = Exclusive Or(1:w140, 2:"Button\n    C") -> (0:w139:bool)
          n155 = Absolute Value(x=w184) -> (abs(x)=w221:dbl)
          n156 = Greater?(x=w225, y=10000.0) -> (0:w223:bool)
          n157 = Greater?(x=w221, y=10000.0) -> (0:w219:bool)
          n158 = case shown="True" w145 {
            tunnel: "Button\n    A" -> [_ w254]
            frame False {
            }
            frame True {
              n159 = call <vilib>:"DIO_PanelSim_Global.vi"("menu"=DIO_Update_Ops."set value", "DIO Channel"=FPGA_DIOChannel."DIO 0", "Value Set"=w254) -> ("DIO new"=→"DIO 0":T5)  [unwired: 11 in, 1 out]
            }
          }
          n160 = case shown="True" w142 {
            tunnel: "Button\n    B" -> [_ w250]
            frame False {
            }
            frame True {
              n161 = call <vilib>:"DIO_PanelSim_Global.vi"("menu"=DIO_Update_Ops."set value", "DIO Channel"=FPGA_DIOChannel."DIO 1", "Value Set"=w250) -> ("DIO new"=→"DIO 1\nIn":T5)  [unwired: 11 in, 1 out]
            }
          }
          n162 = case shown="True" w139 {
            tunnel: "Button\n    C" -> [_ w246]
            frame False {
            }
            frame True {
              n163 = call <vilib>:"DIO_PanelSim_Global.vi"("menu"=DIO_Update_Ops."set value", "DIO Channel"=FPGA_DIOChannel."DIO 2", "Value Set"=w246) -> ("DIO new"=→"DIO 2\nIn":T5)  [unwired: 11 in, 1 out]
            }
          }
          n164 = Build Array(w199) -> (w203:dbl[])
          n165 = Select(t=100000000000000.0, s=w223, f=w183) -> (s? t:f=w217:dbl)
          n166 = Select(t=100000000000000.0, s=w219, f=w184) -> (s? t:f=w216:dbl)
          n167 = call <vilib>:"BatterySim_CalculateLoadedBatteryVoltage.vi"("Currents"=w203, "Resistance_Ohms"=0.3, "NominalVoltage"=w189) -> ("Voltage"=w188:dbl)  [unwired: 8 in]
          "Battery Voltage VDC" <- w188
          n168 = Wait (ms)(milliseconds to wait=u32 20) -> ()  [unwired: 1 out]
          n169 = local read "Stop Sim"() -> (w215:bool)
          n170 = call <vilib>:"Encoder_PanelSim_Global.vi"("menu"=Encoder_Update_Ops."set period", "EncoderIndex"=w164, "Numeric Value"=w217) -> ("error out"=w155:errorcluster)  [unwired: 11 in, 1 out]
          n171 = call <vilib>:"Encoder_PanelSim_Global.vi"("menu"=Encoder_Update_Ops."set count", "EncoderIndex"=w164, "Numeric Value"=w179, "error in (no error)"=w155) -> ("Encoder new"=→"Enc Left":T7)  [unwired: 10 in, 1 out]
          n172 = call <vilib>:"Encoder_PanelSim_Global.vi"("menu"=Encoder_Update_Ops."set period", "EncoderIndex"=w163, "Numeric Value"=w216) -> ("error out"=w153:errorcluster)  [unwired: 11 in, 1 out]
          n173 = call <vilib>:"Encoder_PanelSim_Global.vi"("menu"=Encoder_Update_Ops."set count", "EncoderIndex"=w163, "Numeric Value"=w178, "error in (no error)"=w153) -> ("Encoder new"=→"Enc Right":T7)  [unwired: 10 in, 1 out]
        }
      }
    }
  }
  n174 = while {
    tunnel: w28 -> [_]
    stop <- FALSE stop-if-true
    # "Listen for connection.  When connected process\nmessages with the simulated robot control\nsystem code running on a PC."
    n175 = flat-sequence {
      tunnel: [w275] -> w269
      tunnel: [w273] -> w268
      frame #0 {
        w276 = -1  # timeout ms  (25000)
        w277 = u16 3300  # port
        n176 = local write "Stop Sim"(TRUE ("Stop\nSim")) -> ()
        n177 = call "Robot_Simulation_Connect_Listen.vi"("timeout ms (25000)"=w276, "port"=w277) -> ("error out"=w275:errorcluster, "Properties:Request URI"=→"Request URI":string, "Properties:Return Headers"=→"HTTP Headers":variant, "WebSocket Connection out"=w273:refnum<class "websocket server.lvclass">)  [unwired: 6 in]
      }
    }
    n178 = case shown="No Error" w269 {
      tunnel: w268 -> [w278 _]
      frame No Error {
        n179 = local write "Stop Sim"(FALSE ("Stop\nSim")) -> ()
        n180 = call <vilib>:"WebSocket Server Connection Handler.vi"("WebSocket in"=w278) -> ()  [unwired: 10 in, 1 out]
      }
      frame Error {
      }
    }
  }
